vi "read_master_hbt.vi"(10 "hbt":u16, 11 "node":u8) -> (2 "hbt":u16, 3 "return":i16)   [LabVIEW 2011]
uses:
  canopen_dll_master.dll
panel:
  in  "hbt":cluster{"hbt":u16}
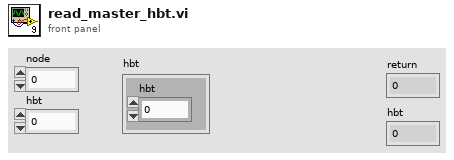
[diagram p1: front panel]
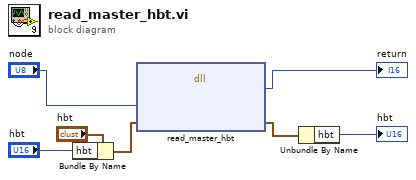
[diagram p0: block diagram]
diagram:
  n1 = Bundle By Name(cluster="hbt", "hbt"="hbt") -> (w3:cluster{"hbt":u16})
  n2 = dll-call lib="canopen_dll_master.dll" fn="read_master_hbt"("node"="node", "hbt"=w3) -> ("return type"=→"return":i16, "hbt"=w2:cluster{"hbt":u16})  [unwired: 4 in, 2 out]
  n3 = Unbundle By Name(w2) -> ("hbt"=→"hbt":u16)
